vi "Initialization VI.vi"(8 "error in (no error)":errorcluster, 10 "Custom XML":string, 11 "Device Item Ref in":T1 format="%.0x") -> (0 "error out":errorcluster, 3 "Device Item Ref out":T1 format="%.0x")   [LabVIEW 2024, in "Embedded TDMS Logger System Explorer.lvlib"]
doc: "Initialization VI called when the custom device is created - unchanged from the original template creation by the Custom Device Development Tool Wizard except the deletion of the query to the user about a new device instance or a copy."
uses:
  Embedded TDMS Logger System Explorer.lvlib
  <vilib>/NI VeriStand/Custom Device API/Custom Device Item Ref.ctl
  <vilib>/NI VeriStand/Custom Device API/Set Item Property (U16).vi
  <vilib>/NI VeriStand/Custom Device API/Custom Device API.lvlib
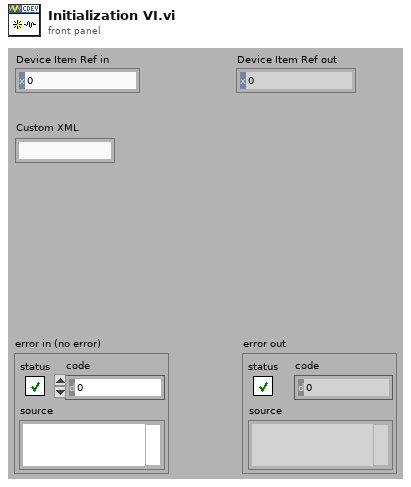
[diagram p1: front panel]
types:
  T1 = typedef "Custom Device API.lvlib/Custom Device Item Ref.ctl" = u64
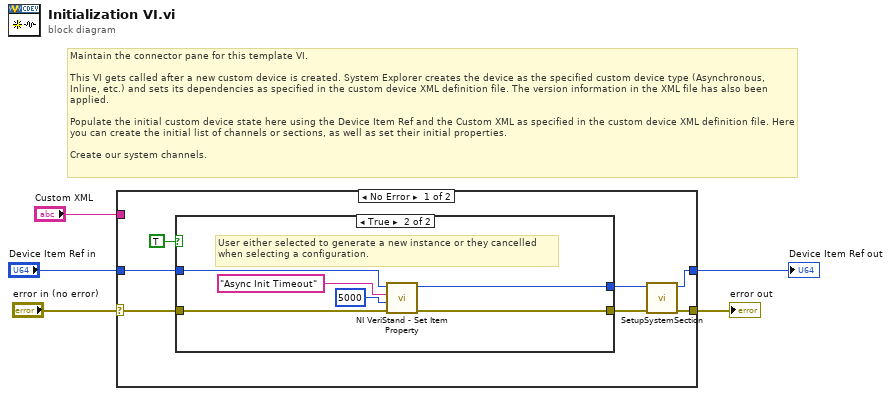
[diagram p0: block diagram]
diagram:
  # "Maintain the connector pane for this template VI.\n\nThis VI gets called after a new custom device is created. System Explorer creates the device as the specified custom device type (Asynchronous, Inline, etc.) and sets its dependencies as specified in the custom device XML definition file. The version information in the XML file has also been applied.\n\nPopulate the initial custom device state here using the Device Item Ref and the Custom XML as specified in the custom device XML definition file. Here you can create the initial list of channels or sections, as well as set their initial properties.\n\nCreate our system channels."
  n1 = case shown="No Error" "error in (no error)" {
    selector: "error in (no error)" -> [w10 w22]
    tunnel: [w7 w22] -> w5
    tunnel: [w8 w21] -> w3
    tunnel: "Device Item Ref in" -> [w11 w21]
    tunnel: "Custom XML" -> [_ _]
    frame No Error {
      n2 = case "Create New" shown="True" TRUE {
        tunnel: w11 -> [w14 w18]
        tunnel: w10 -> [w13 w19]
        tunnel: [w13 w17] -> w6
        tunnel: [w14 w16] -> w9
        frame False {
          # "User selected to import from configuration and didn't cancel import"
        }
        frame True {
          # "User either selected to generate a new instance or they cancelled\nwhen selecting a configuration."
          n3 = call-poly <vilib>:"NI VeriStand - Set Item Property.vi"("error in (no error)"=w19, "Value"=u16 5000, "Property Name"="Async Init Timeout", "Item Ref in"=w18) -> ("error out"=w17:errorcluster, "Item Ref out"=w16:T1)  [unwired: 5 in, 1 out]
        }
      }
      n4 = call "SetupSystemSection.vi"("error in (no error)"=w6, "Node Ptr"=w9) -> ("error out"=w7:errorcluster, "Parent Ref Out"=w8:T1)  [unwired: 5 in, 3 out]
    }
    frame Error {
    }
  }
  "error out" <- w5
  "Device Item Ref out" <- w3
